vi "Filter Levels.vi"(7 "Decay":dbl, 10 "Levels In":dbl[](array[numeric])) -> (2 "Fitlered Levels":dbl[](array[numeric]))   [LabVIEW 2022 SP3, in "TouchControl.lvlib" / "AudioMonPanel.lvclass"]
uses:
  AudioMonPanel.lvclass
  AudioMonPanel.lvclass/AudioMonPanel.ctl
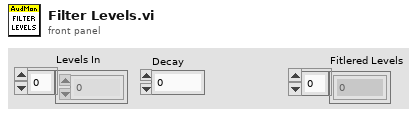
[diagram p1: front panel]
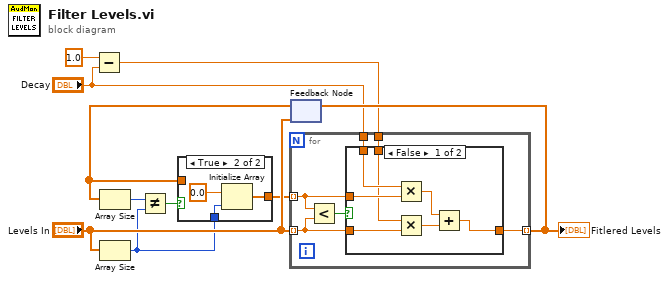
[diagram p0: block diagram]
diagram:
  n1 = Subtract(x=1.0, y="Decay") -> (x-y=w2:dbl)
  n2 = Array Size(array="Levels In") -> (size(s)=w7:i32)
  n3 = feedback #1("Levels In") -> (w5:dbl[])
  n4 = Array Size(array=w5) -> (size(s)=w9:i32)
  n5 = Not Equal?(x=w9, y=w7) -> (x != y?=w8:bool)
  n6 = case shown="True" w8 {
    tunnel: w7 -> [_ w14]
    tunnel: [w11 w12] -> w6
    tunnel: w5 -> [w11 _]
    frame False {
    }
    frame True {
      n7 = Initialize Array(0.0 ("element"), w14) -> (w12:dbl[])
    }
  }
  n8 = for {
    tunnel: "Levels In" -> [w20] mode=indexing
    tunnel: w6 -> [w18] mode=indexing
    tunnel: [w17] -> w4 mode=indexing
    tunnel: w2 -> [w16]
    tunnel: "Decay" -> [w15]
    n9 = Less?(x=w18, y=w20) -> (x < y?=w19:bool)
    n10 = case shown="False" w19 {
      tunnel: w20 -> [w25 w28]
      tunnel: w18 -> [w26 _]
      tunnel: [w21 w28] -> w17
      tunnel: w16 -> [w24 _]
      tunnel: w15 -> [w27 _]
      frame False {
        n11 = Multiply(x=w27, y=w26) -> (x*y=w22:dbl)
        n12 = Multiply(x=w24, y=w25) -> (x*y=w23:dbl)
        n13 = Add(x=w22, y=w23) -> (x+y=w21:dbl)
      }
      frame True {
      }
    }
  }
  "Fitlered Levels" <- w4
  n14 = feedback-in #1(w4) -> ()
